vi "catch_block_in_body_test.vi"() -> ()   [LabVIEW 2013]
panel:
  out "Voltage":dbl(graph)
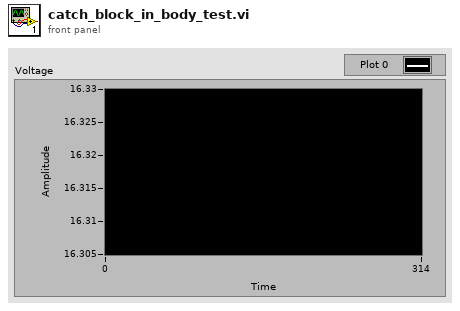
[diagram p1: front panel]
types:
  T1 = typedef "KNR3 Reference.ctl" = cluster{"FPGA Session":refnum<class "FPGA Interface Base.lvclass">, "Resource":T2}
  T2 = typedef "Resource.ctl" = enum16{"KNRm_DDRC", "KNRm_DDDD", "KNRm_DDDR", "KNRm_DDDC", "KNR"}
  T3 = cluster{"Mode":enum16{"FRWD", "TURFIX", "TURNOF"}, "Dir":enum16{"Left", "Right"}, "Pcmd":dbl, "Vcmd":dbl}
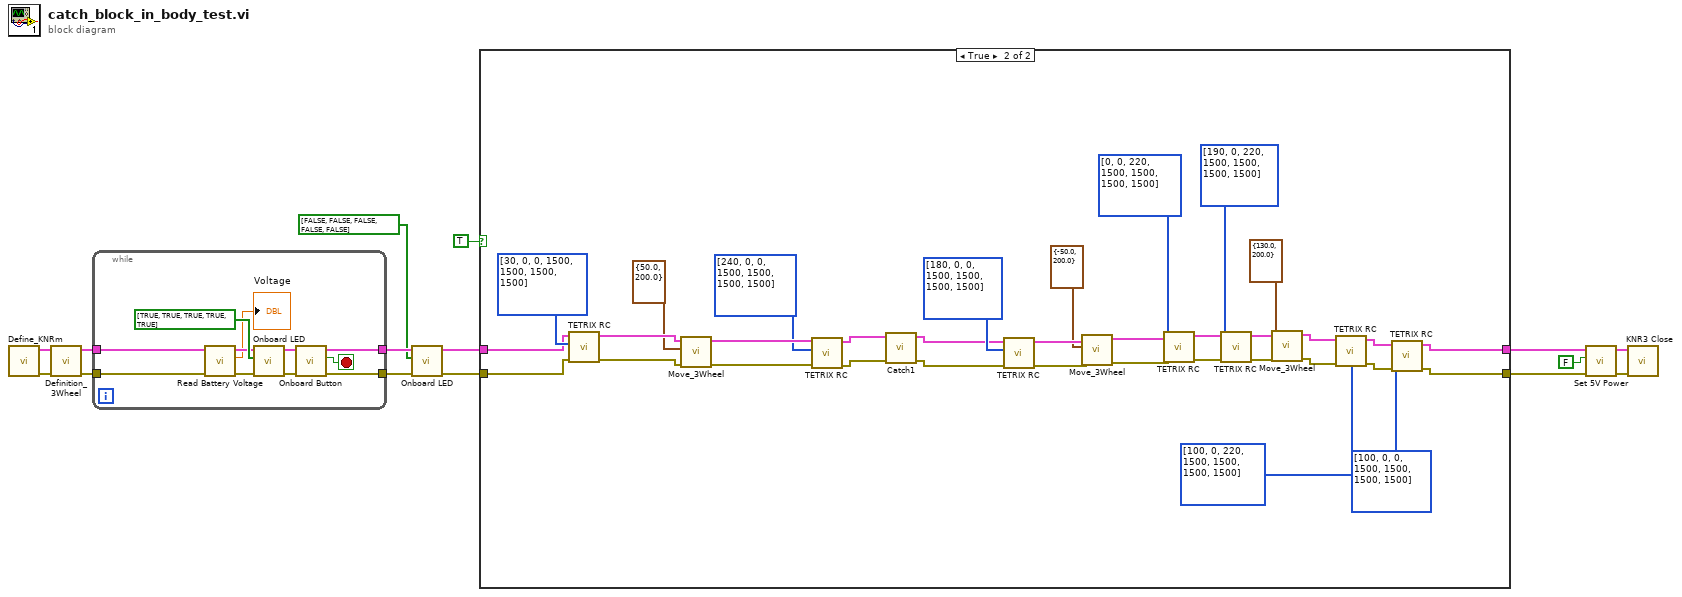
[diagram p0: block diagram]
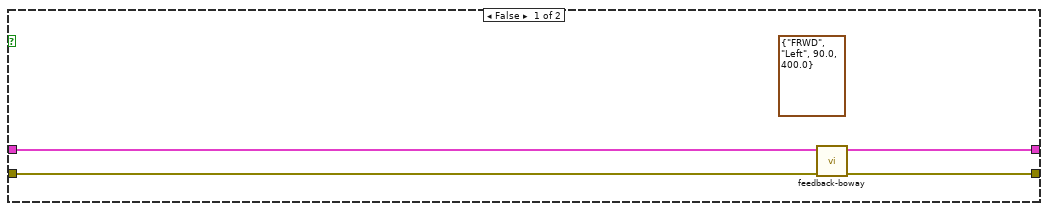
[diagram p2: hidden frame]
diagram:
  n1 = call "Define_KNRm.vi"() -> ("error out"=w6:errorcluster, "KNR out"=w7:T1)  [unwired: 10 in]
  n2 = call "Definition_3Wheel.vi"("error in (no error)"=w6, "KNR in"=w7) -> ("error out"=w8:errorcluster, "KNR out"=w9:T1)  [unwired: 8 in]
  n3 = while {
    tunnel: [w25] -> w15
    tunnel: [w23] -> w13
    tunnel: w9 -> [w18]
    tunnel: w8 -> [w17]
    stop <- w26 stop-if-true
    n4 = call <userlib>:"Read Battery Voltage.vi"("error in (no error)"=w17, "KNR in"=w18) -> ("error out"=w19:errorcluster, "Voltage"=→"Voltage":dbl, "KNR out"=w20:T1)  [unwired: 7 in]
    n5 = call <userlib>:"Onboard LED.vi"("error in (no error)"=w19, "LED List"=bool[] [TRUE, TRUE, TRUE, TRUE, TRUE], "KNR in"=w20) -> ("error out"=w24:errorcluster, "KNR out"=w22:T1)  [unwired: 7 in]
    n6 = call <userlib>:"Onboard Button.vi"("error in (no error)"=w24, "KNR in"=w22) -> ("error out"=w23:errorcluster, "value"=w26:bool, "KNR out"=w25:T1)  [unwired: 7 in]
  }
  n7 = call <userlib>:"Onboard LED.vi"("error in (no error)"=w13, "LED List"=bool[] [FALSE, FALSE, FALSE, FALSE, FALSE], "KNR in"=w15) -> ("error out"=w10:errorcluster, "KNR out"=w11:T1)  [unwired: 7 in]
  n8 = case shown="True" TRUE {
    tunnel: w10 -> [w30 w62]
    tunnel: [w29 w31] -> w1
    tunnel: w11 -> [w28 w63]
    tunnel: [w27 w32] -> w2
    frame False {
      (unwired) T3 {"Mode"=enum."FRWD", "Dir"=enum."Left", "Pcmd"=90.0, "Vcmd"=400.0} ("Move")
      n9 = call "feedback-boway.vi"("error in (no error)"=w30, "KNR in"=w28) -> ("error out"=w29:errorcluster, "KNR out"=w27:T1)  [unwired: 7 in, 1 out]
    }
    frame True {
      n10 = call "TETRIX RC.vi"("error in 2"=w62, "RC"=u16[] [30, 0, 0, 1500, 1500, 1500, 1500], "KNR in 3"=w63) -> ("error out 4"=w60:errorcluster, "KNR out 4"=w61:T1)  [unwired: 7 in]
      n11 = call "Move_3Wheel.vi"("error in (no error)"=w60, "Cluster"=cluster{"UDmm)":dbl, "Vcmd":dbl} {"UDmm)"=50.0, "Vcmd"=200.0}, "KNR in"=w61) -> ("error out"=w57:errorcluster, "KNR out"=w58:T1)  [unwired: 7 in]
      n12 = call "TETRIX RC.vi"("error in 2"=w57, "RC"=u16[] [240, 0, 0, 1500, 1500, 1500, 1500], "KNR in 3"=w58) -> ("error out 4"=w41:errorcluster, "KNR out 4"=w42:T1)  [unwired: 7 in]
      n13 = call "Catch1.vi"("Error"=w41, "KNR in"=w42) -> ("error out 4"=w39:errorcluster, "KNR out"=w40:T1)  [unwired: 6 in, 2 out]
      n14 = call "TETRIX RC.vi"("error in 2"=w39, "RC"=u16[] [180, 0, 0, 1500, 1500, 1500, 1500], "KNR in 3"=w40) -> ("error out 4"=w53:errorcluster, "KNR out 4"=w54:T1)  [unwired: 7 in]
      n15 = call "Move_3Wheel.vi"("error in (no error)"=w53, "Cluster"=cluster{"UDmm)":dbl, "Vcmd":dbl} {"UDmm)"=-50.0, "Vcmd"=200.0}, "KNR in"=w54) -> ("error out"=w50:errorcluster, "KNR out"=w51:T1)  [unwired: 7 in]
      n16 = call "TETRIX RC.vi"("error in 2"=w50, "RC"=u16[] [0, 0, 220, 1500, 1500, 1500, 1500], "KNR in 3"=w51) -> ("error out 4"=w47:errorcluster, "KNR out 4"=w48:T1)  [unwired: 7 in]
      n17 = call "TETRIX RC.vi"("error in 2"=w47, "RC"=u16[] [190, 0, 220, 1500, 1500, 1500, 1500], "KNR in 3"=w48) -> ("error out 4"=w45:errorcluster, "KNR out 4"=w44:T1)  [unwired: 7 in]
      n18 = call "Move_3Wheel.vi"("error in (no error)"=w45, "Cluster"=cluster{"UDmm)":dbl, "Vcmd":dbl} {"UDmm)"=130.0, "Vcmd"=200.0}, "KNR in"=w44) -> ("error out"=w37:errorcluster, "KNR out"=w38:T1)  [unwired: 7 in]
      n19 = call "TETRIX RC.vi"("error in 2"=w37, "RC"=u16[] [100, 0, 220, 1500, 1500, 1500, 1500], "KNR in 3"=w38) -> ("error out 4"=w35:errorcluster, "KNR out 4"=w34:T1)  [unwired: 7 in]
      n20 = call "TETRIX RC.vi"("error in 2"=w35, "RC"=u16[] [100, 0, 0, 1500, 1500, 1500, 1500], "KNR in 3"=w34) -> ("error out 4"=w31:errorcluster, "KNR out 4"=w32:T1)  [unwired: 7 in]
    }
  }
  n21 = call <userlib>:"Set 5V Power.vi"("error in (no error)"=w1, "5V Power(T)"=FALSE, "KNR in"=w2) -> ("error out"=w4:errorcluster, "KNR out"=w5:T1)  [unwired: 7 in]
  n22 = call <userlib>:"KNR3 Close.vi"("error in (no error)"=w4, "KNR in"=w5) -> ()  [unwired: 9 in, 1 out]
